vi "To Waveform.vi"(8 "error in (no error)":errorcluster, 11 "Waveform in":refnum<class "Waveform.lvclass">) -> (0 "error out":errorcluster, 1 "Success?":bool, 3 "Waveform Array":waveform(dbl)[](array[waveform]))   [LabVIEW 2020, in "Data.lvlib" / "Waveform.lvclass"]
doc: "Interpret 'Data' as a Waveform Array. If impossible 'Success?' is set to FALSE"
uses:
  Waveform.lvclass
  Waveform.lvclass/Waveform.ctl
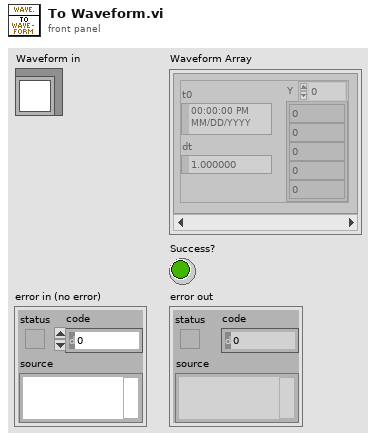
[diagram p1: front panel]
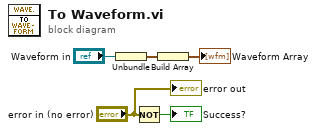
[diagram p0: block diagram]
diagram:
  n1 = Unbundle("Waveform in") -> (w4:waveform(dbl))
  n2 = Not(x="error in (no error)") -> (.not. x?=→"Success?":bool)
  n3 = Build Array(w4) -> (→"Waveform Array":waveform(dbl)[])
  "error out" <- "error in (no error)"
